vi "Traditional UI.vi"(11 "Process in":refnum<class "ABD.lvclass">) -> (0 "error out":errorcluster, 3 "Process out":refnum<class "ABD.lvclass">)   [LabVIEW 2021, in "ABD.lvlib" / "ABD.lvclass"]
uses:
  ABD.lvclass
  ABD.lvclass/ABD.ctl
  LVCAM/Msgs/LVCAM Destroy Self/LVCAM Destroy Self Msg/LVCAM Destroy Self Msg.lvclass
  C:/PPLs/LabVIEW-Composed-Actor-Model-LVCAM/LabVIEW-Composed-Actor-Model-LVCAM/LVCAM/LVCAM/Msg/Msg.lvclass
  LVCAM/LVCAM/Self Actor/Self Msg Send.vi
  LVCAM/LVCAM/Self Actor/Self Actor.lvclass
  C:/PPLs/LabVIEW-Composed-Actor-Model-LVCAM/LabVIEW-Composed-Actor-Model-LVCAM/LVCAM/Msgs/LVCAM Destroy Self/LVCAM Destroy Self Msg/LVCAM Destroy Self Msg.lvclass
  C:/PPLs/LabVIEW-Composed-Actor-Model-LVCAM/LabVIEW-Composed-Actor-Model-LVCAM/LVCAM/Msgs/LVCAM Destroy Self/LVCAM Destroy Self/LVCAM Destroy Self.lvclass
panel:
  # "PANEL"
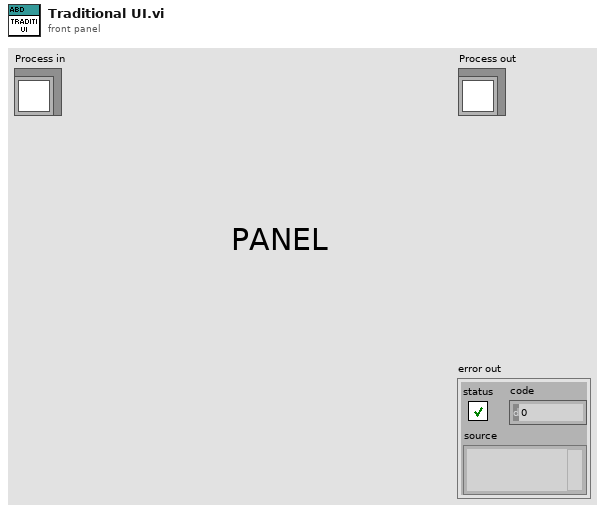
[diagram p1: front panel]
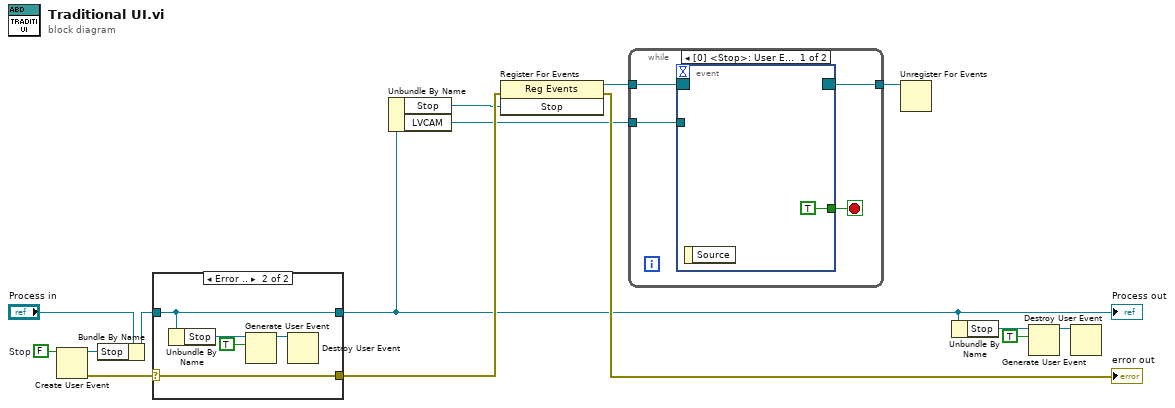
[diagram p0: block diagram]
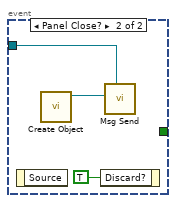
[diagram p2: hidden frame]
diagram:
  w13 = FALSE  # Stop
  n1 = Create User Event(user event datatype=w13) -> (user event=w14:refnum<user-event>, error out=w12:errorcluster)  [unwired: 1 in]
  n2 = Bundle By Name(cluster="Process in", "Stop"=w14) -> (w11:refnum<class "ABD.lvclass">)
  n3 = case shown="Error .." w12 {
    selector: w12 -> [_ w21]
    tunnel: [w16 w17] -> w2
    tunnel: w11 -> [w16 w17]
    tunnel: [_ w21] -> w7
    frame No Error {
    }
    frame Error {
      n4 = Unbundle By Name(w17) -> ("Stop"=w18:refnum<user-event>)
      n5 = Generate User Event(user event=w18, event data cluster=TRUE ("event data")) -> (user event out=w19:refnum<user-event>)  [unwired: 2 in, 1 out]
      n6 = Destroy User Event(user event=w19) -> ()  [unwired: 1 in, 1 out]
    }
  }
  "Process out" <- w2
  n7 = Unbundle By Name(w2) -> ("Stop"=w6:refnum<user-event>, "LVCAM"=w1:refnum<class "LVCAM.lvclass">)
  n8 = register-events ("Main Register for Events")(error in=w7, w6) -> (reference out=w10:refnum<event-registration>, error out=→"error out":errorcluster)  [unwired: 1 in]
  n9 = while {
    tunnel: w10 -> [w25]
    tunnel: [w23] -> w9
    tunnel: w1 -> [w22]
    stop <- w24 stop-if-true
    n10 = event "UI Events" shown="[0] <Stop>: User Event" {
      selector: w25 -> [_ _]
      dyn-events: [_ _] -> w23
      timeout: _ -> [_ _]
      tunnel: [TRUE _] -> w24
      tunnel: w22 -> [_ w28]
      event User Event {
        n11 = event-data() -> ()  [unwired: 1 in, 1 out]
      }
      event Panel Close? {
        n12 = event-data() -> ()  [unwired: 1 in, 1 out]
        n13 = call "Create Object.vi"() -> ("LVCAM Destroy Self Msg out"=w27:refnum<class "LVCAM Destroy Self Msg.lvclass">)  [unwired: 11 in]
        n14 = event-data("Discard?"=TRUE) -> ()  [unwired: 1 in, 1 out]
        n15 = call-poly "Msg Send.vi"("Self Actor"=w28, "Msg"=w27) -> ()  [unwired: 9 in, 1 out]
      }
    }
  }
  n16 = Unregister For Events(event registration refnum=w9) -> ()  [unwired: 1 in, 1 out]
  n17 = Unbundle By Name(w2) -> ("Stop"=w5:refnum<user-event>)
  n18 = Generate User Event(user event=w5, event data cluster=TRUE ("event data")) -> (user event out=w4:refnum<user-event>)  [unwired: 2 in, 1 out]
  n19 = Destroy User Event(user event=w4) -> ()  [unwired: 1 in, 1 out]
